vi "Lookup Channel Indices.vi"(8 "error in (no error)":errorcluster, 11 "Log Manager Module in":refnum<class "Log Manager Module.lvclass">) -> (0 "error out":errorcluster, 3 "Log Manager Module out":refnum<class "Log Manager Module.lvclass">)   [LabVIEW 2020, in "VolatusData.lvlib" / "Log Manager Module.lvclass"]
uses:
  Log Manager Module.lvclass
  C:/dev/lv20CE/relink/lv-volatus/Volatus/Module/Module.lvclass
  VolatusConfig/Meta Type.ctl
  Log Manager Module.lvclass/Log Manager Module.ctl
  Volatus/Module/Module.lvclass/Module.ctl
  VolatusConfig/VolatusConfigElement/VolatusConfigElement.lvclass/VolatusConfigElement.ctl
  VolatusConfig/VolatusConfigElement/Element.vi
  VolatusConfig/Channel/Channel Config.lvclass
  C:/dev/lv20CE/relink/lv-volatus/VolatusConfig/VolatusConfigElement/VolatusConfigElement.lvclass
  lv-vecto/Vecto/Group STR/Group STR.lvclass
  C:/dev/lv20CE/relink/lv-vecto/Vecto/Group/Group.lvclass
  lv-cdm/CDM-Config/Config Lookup/Match Meta.vi
  lv-cdm/CDM-Config/Config Element/Owner.vi
  lv-cdm/CDM-Config/Config Manager/Lookup Descendant.vi
  lv-cdm/CDM-Config/Config Filter/Config Lookup.lvclass
  Volatus/Module/Module.lvclass
  VolatusConfig/VolatusConfig.lvlib
  VolatusConfig/VolatusConfigElement/VolatusConfigElement.lvclass
  VolatusConfig/Group/Group Config.lvclass
  lv-vecto/Vecto/Group/Group.lvclass
  C:/dev/lv20CE/relink/lv-volatus/VolatusData/Log Manager Module/Log Manager Module.lvclass
  C:/dev/lv20CE/relink/lv-volatus/VolatusConfig/Channel/Channel Config.lvclass
  lv-vecto/Vecto/Group DBL/Group DBL.lvclass
  C:/dev/lv20CE/relink/lv-vecto/Vecto/Group DBL/Group DBL.lvclass
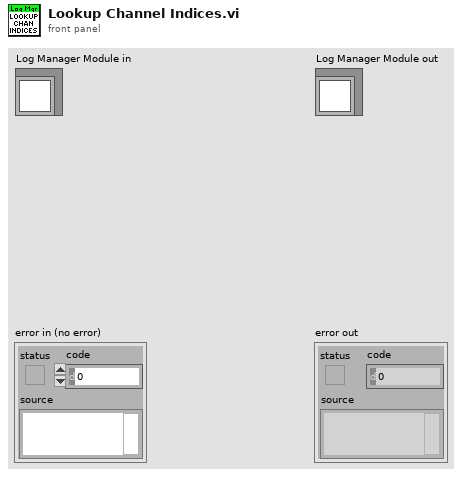
[diagram p1: front panel]
types:
  T1 = typedef "VolatusConfig.lvlib/Meta Type.ctl" = enum16{"UNKNOWN", "VL_System", "VL_Cluster", "VL_Node", "VL_Task", "VL_Group", "VL_Channel", "VL_Task_List", "VL_Scaling", "VL_Sensor", "VL_Sensor_List", "VL_Scale"}
  T2 = typedef "VectoConfig.lvlib/Channel Info.ctl" = cluster{"Name":string, "Group":string, "Owning Node":string, "Owning Task":string, "Resource":string}
  T3 = typedef "VolatusData.lvlib/Log Manager Module.lvclass/Channel Indices.ctl" = cluster{"State_Num":i32, "Num_Loggers":i32, "Num_Idle":i32, "Num_Prep":i32, "Num_Ready":i32, "Num_Active":i32, "Num_Stopping":i32, "All_Active":i32}
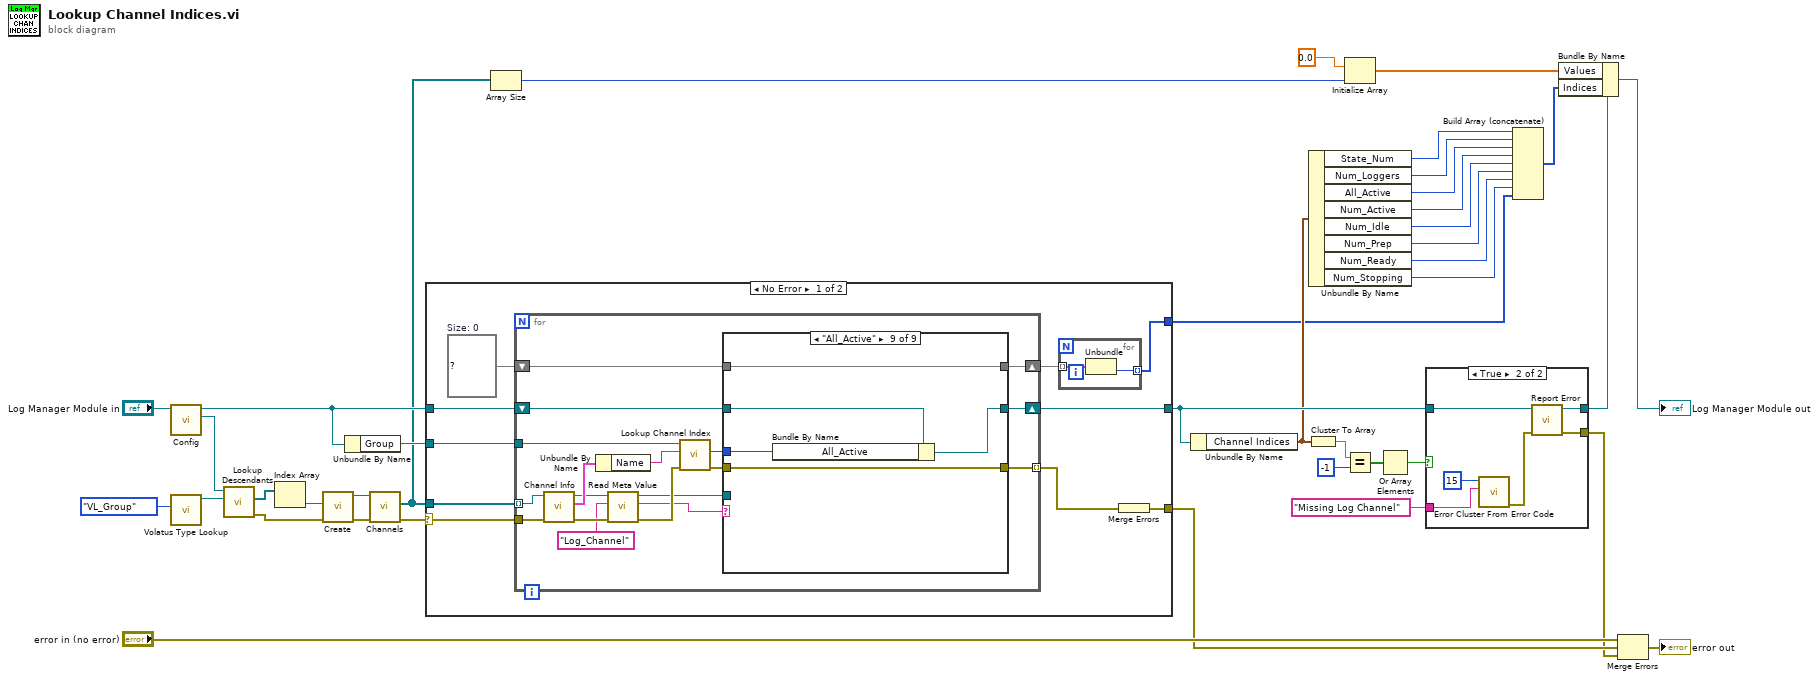
[diagram p0: block diagram]
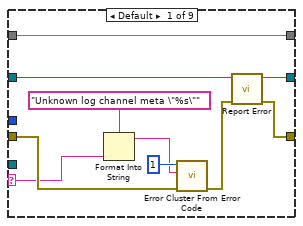
[diagram p2: hidden frame]
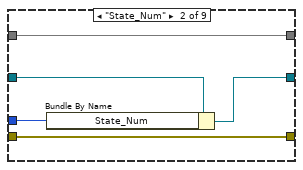
[diagram p3: hidden frame]
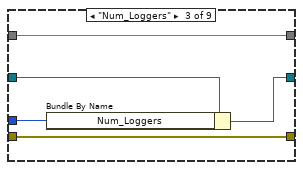
[diagram p4: hidden frame]
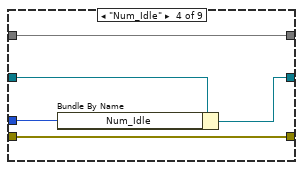
[diagram p5: hidden frame]
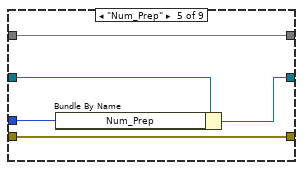
[diagram p6: hidden frame]
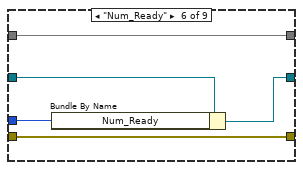
[diagram p7: hidden frame]
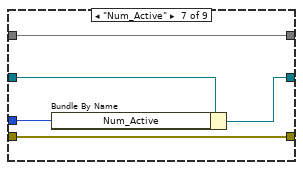
[diagram p8: hidden frame]
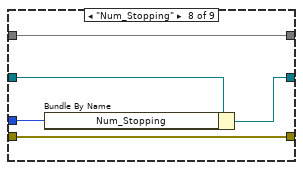
[diagram p9: hidden frame]
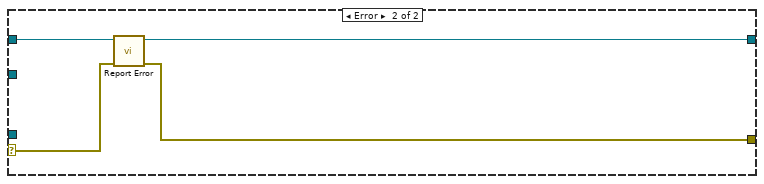
[diagram p10: hidden frame]
diagram:
  n1 = call "Config.vi"("Module in"="Log Manager Module in") -> ("Config"=w36:refnum<class "VolatusConfigElement.lvclass">, "Module out"=w28:refnum<class "Log Manager Module.lvclass">)  [unwired: 9 in]
  n2 = call "Volatus Type Lookup.vi"("Meta Type"=Meta_Type."VL_Group") -> ("Config Lookup out"=w35:refnum<class "Config Lookup.lvclass">)  [unwired: 9 in, 1 out]
  n3 = call "Lookup Descendants.vi"("Lookup"=w35, "VolatusConfigElement in"=w36) -> ("error out"=w30:errorcluster, "Descendants"=w34:refnum<class "Config Element.lvclass">[])  [unwired: 7 in, 1 out]
  n4 = Index Array(array=w34) -> (element=w33:refnum<class "Config Element.lvclass">)  [unwired: 1 in]
  n5 = call "Create.vi"("error in (no error)"=w30, "Element"=w33) -> ("error out"=w31:errorcluster, "Group out"=w32:refnum<class "Group Config.lvclass">)  [unwired: 8 in]
  n6 = Unbundle By Name(w28) -> ("Group"=w29:refnum<class "Group DBL.lvclass">)
  n7 = call "Channels.vi"("error in (no error)"=w31, "Group in"=w32) -> ("error out"=w27:errorcluster, "Channels"=w4:refnum<class "Channel Config.lvclass">[])  [unwired: 7 in, 1 out]
  n8 = case shown="No Error" w27 {
    selector: w27 -> [w46 w122]
    tunnel: w29 -> [w49 _]
    tunnel: w28 -> [w48 w123]
    tunnel: w4 -> [w47 _]
    tunnel: [w40 w121] -> w22
    tunnel: [w44 w120] -> w19
    tunnel: [w41 _] -> w1
    frame No Error {
      w43 = map{string, i32} {}  # Size: 0
      n9 = for {
        tunnel: w49 -> [w65]
        shift-right: [w56] -> w40
        shift-left: w48 -> [w59]
        tunnel: w47 -> [w68] mode=indexing
        tunnel: w46 -> [w67]
        tunnel: [w55] -> w45 mode=indexing
        shift-right: [w52] -> w42
        shift-left: w43 -> [w53]
        n10 = call "Channel Info.vi"("error in (no error)"=w67, "Channel in"=w68) -> ("error out"=w62:errorcluster, "Channel Info"=w66:T2, "Channel out"=w63:refnum<class "Channel Config.lvclass">)  [unwired: 7 in]
        n11 = Unbundle By Name(w66) -> ("Name"=w64:string)
        n12 = call "Read Meta Value.vi"("error in (no error)"=w62, "Meta Name"="Log_Channel", "VolatusConfigElement in"=w63) -> ("error out"=w69:errorcluster, "Meta Value"=w58:string, "VolatusConfigElement out"=w54:refnum<class "Channel Config.lvclass">)  [unwired: 6 in]
        n13 = call "Lookup Channel Index.vi"("error in (no error)"=w69, "Channel Name"=w64, "Group in"=w65) -> ("error out"=w57:errorcluster, "Index"=w60:i32)  [unwired: 6 in, 1 out]
        n14 = case shown="\"All_Active\"" w58 {
          selector: w58 -> [w76 _ _ _ _ _ _ _ _]
          tunnel: w60 -> [_ w83 w88 w93 w98 w103 w108 w113 w118]
          tunnel: w59 -> [w74 w84 w89 w94 w99 w104 w109 w114 w119]
          tunnel: w57 -> [w78 w81 w86 w91 w96 w101 w106 w111 w116]
          tunnel: [w73 w82 w87 w92 w97 w102 w107 w112 w117] -> w56
          tunnel: [w71 w81 w86 w91 w96 w101 w106 w111 w116] -> w55
          tunnel: w54 -> [_ _ _ _ _ _ _ _ _]
          tunnel: w53 -> [w70 w80 w85 w90 w95 w100 w105 w110 w115]
          tunnel: [w70 w80 w85 w90 w95 w100 w105 w110 w115] -> w52
          frame Default {
            n15 = Format Into String(format string="Unknown log channel meta \"%s\"", w76) -> (resulting string=w75:string)  [unwired: 2 in, 1 out]
            n16 = call <vilib>:"Error Cluster From Error Code.vi"("error in (no error)"=w78, "error message (\"\")"=w75, "error code (0)"=1) -> ("error out"=w72:errorcluster)  [unwired: 6 in]
            n17 = call "Report Error.vi"("error in (no error)"=w72, "Module in"=w74) -> ("error out"=w71:errorcluster, "Module out"=w73:refnum<class "Log Manager Module.lvclass">)  [unwired: 8 in]
          }
          frame "State_Num" {
            n18 = Bundle By Name(cluster=w84, "State_Num"=w83) -> (w82:refnum<class "Log Manager Module.lvclass">)
          }
          frame "Num_Loggers" {
            n19 = Bundle By Name(cluster=w89, "Num_Loggers"=w88) -> (w87:refnum<class "Log Manager Module.lvclass">)
          }
          frame "Num_Idle" {
            n20 = Bundle By Name(cluster=w94, "Num_Idle"=w93) -> (w92:refnum<class "Log Manager Module.lvclass">)
          }
          frame "Num_Prep" {
            n21 = Bundle By Name(cluster=w99, "Num_Prep"=w98) -> (w97:refnum<class "Log Manager Module.lvclass">)
          }
          frame "Num_Ready" {
            n22 = Bundle By Name(cluster=w104, "Num_Ready"=w103) -> (w102:refnum<class "Log Manager Module.lvclass">)
          }
          frame "Num_Active" {
            n23 = Bundle By Name(cluster=w109, "Num_Active"=w108) -> (w107:refnum<class "Log Manager Module.lvclass">)
          }
          frame "Num_Stopping" {
            n24 = Bundle By Name(cluster=w114, "Num_Stopping"=w113) -> (w112:refnum<class "Log Manager Module.lvclass">)
          }
          frame "All_Active" {
            n25 = Bundle By Name(cluster=w119, "All_Active"=w118) -> (w117:refnum<class "Log Manager Module.lvclass">)
          }
        }
      }
      n26 = for {
        tunnel: w42 -> [w51] mode=indexing
        tunnel: [w50] -> w41 mode=indexing
        n27 = Unbundle(w51) -> (w50:i32)  [unwired: 1 out]
      }
      n28 = Merge Errors(w45) -> (w44:errorcluster)
    }
    frame Error {
      n29 = call "Report Error.vi"("error in (no error)"=w122, "Module in"=w123) -> ("error out"=w120:errorcluster, "Module out"=w121:refnum<class "Log Manager Module.lvclass">)  [unwired: 8 in]
    }
  }
  n30 = Array Size(array=w4) -> (size(s)=w3:i32)
  n31 = Unbundle By Name(w22) -> ("Channel Indices"=w8:T3)
  n32 = Cluster To Array(cluster=w8) -> (array=w26:i32[])
  n33 = Unbundle By Name(w8) -> ("State_Num"=w16:i32, "Num_Loggers"=w15:i32, "All_Active"=w14:i32, "Num_Active"=w13:i32, "Num_Idle"=w12:i32, "Num_Prep"=w11:i32, "Num_Ready"=w10:i32, "Num_Stopping"=w9:i32)
  n34 = Initialize Array(0.0, w3) -> (w2:dbl[])
  n35 = Equal?(x=w26, y=-1) -> (x = y?=w24:bool[])
  n36 = Or Array Elements(Boolean array=w24) -> (logical OR=w23:bool)
  n37 = case shown="True" w23 {
    tunnel: w22 -> [w124 w130]
    tunnel: [w124 w129] -> w21
    tunnel: [_ w128] -> w18
    tunnel: "Missing Log Channel" -> [_ w125]
    frame False {
    }
    frame True {
      n38 = call <vilib>:"Error Cluster From Error Code.vi"("error message (\"\")"=w125, "error code (0)"=15) -> ("error out"=w126:errorcluster)  [unwired: 7 in]
      n39 = call "Report Error.vi"("error in (no error)"=w126, "Module in"=w130) -> ("error out"=w128:errorcluster, "Module out"=w129:refnum<class "Log Manager Module.lvclass">)  [unwired: 8 in]
    }
  }
  n40 = Build Array (concatenate)(w16, w15, w14, w13, w12, w11, w10, w9, w1) -> (w6:i32[])
  n41 = Bundle By Name(cluster=w21, "Values"=w2, "Indices"=w6) -> (→"Log Manager Module out":refnum<class "Log Manager Module.lvclass">)
  n42 = Merge Errors("error in (no error)", w19, w18) -> (→"error out":errorcluster)
